vi "ief_read_data.vi"(0 "Tagprefix in":refnum<k21>, 11 "error in (no error)":errorcluster) -> (3 "PA Control Error":bool=TRUE, 4 "Tagprefix out":refnum<k21>, 6 "value real 32":sgl format="%.5f", 8 "value uint 32":u32, 10 "value uint 16":u16, 14 "PA Control state":u8, 15 "error out (no error)":errorcluster)   [LabVIEW 2015, in "IEF Werner.lvlib"]
doc: "This VI reads the input bytes from the IEF control and the PA status. \n\nNote that the tags of the DSC engine used by this VI have a strict name convention. This convention is described in the documentation of the VI tree.\n\nLicense Agreement for this software:\n\nCopyright (C)\nGesellschaft für Schwerionenforschung, GSI\nPlanckstr. 1\n64291 Darmstadt\nGermany\n\nContact: D.Beck@gsi.de \n\nThis program is free software; you can redistribute it and/or modify it under the terms of the \nGNU General Public License as published by the Free Software Foundation; either version 2 of \nthe license, or (at your option) any later version.\n\nThis program is distributed in the hope that it will be useful, but WITHOUT ANY WARRANTY; \nwithout even the implied warranty of MERCHANTABILITY or FITNESS FOR A PARTICULAR PURPOSE. See \nthe GNU General License for more details (http://www.gnu.org).\n\nGesellschaft für Schwerionenforschung, GSI\nPlanckstr. 1, 64291 Darmstadt, Germany\nFor all questions and ideas contact: M.Richter@gsi.de, H.Brand@gsi.de or D.Beck@gsi.de.\nLast update: 20-DEC-2002"
uses:
  IEF Werner.lvlib
  Packages/CSPP_Core/Libraries/Base/FGV Action.ctl
  <vilib>/lvdsc/legacy/tag/legacy_Read_Tag_(analog)7x.vi
  Packages/CSPP_Core/Libraries/Base/CS++Base.lvlib
panel:
  # "IEF Read Data"
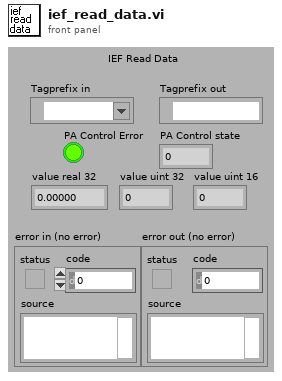
[diagram p1: front panel]
types:
  T1 = typedef "CS++Base.lvlib/FGV Action.ctl" = enum16{"add", "replace", "read", "remove", "reset", "get attributes"}
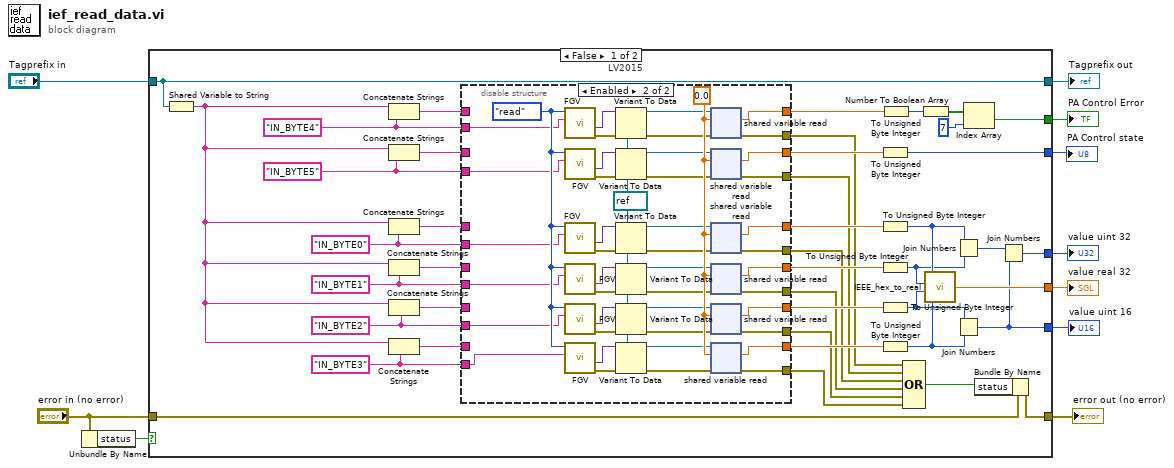
[diagram p0: block diagram]
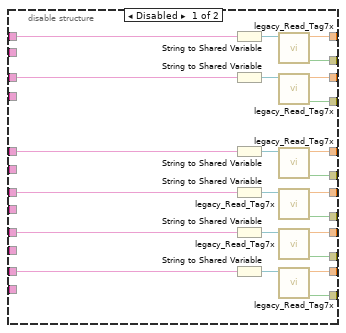
[diagram p2: hidden frame]
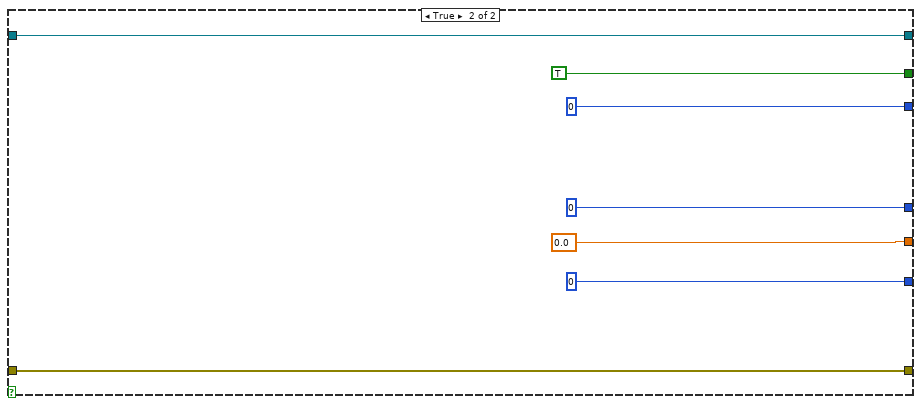
[diagram p3: hidden frame]
diagram:
  n1 = Unbundle By Name("error in (no error)") -> ("status"=w5:bool)
  n2 = case shown="False" w5 {
    tunnel: [w38 sgl 0.0 ("number 5")] -> w10
    tunnel: [w37 u32 0] -> w9
    tunnel: [w36 TRUE] -> w8
    tunnel: [w35 u8 0] -> w7
    tunnel: [w28 u16 0] -> w6
    tunnel: "error in (no error)" -> [w27 w123]
    tunnel: [w26 w123] -> w3
    tunnel: "Tagprefix in" -> [w17 w122]
    tunnel: [w17 w122] -> w1
    frame False {
      w11 = "IN_BYTE3" ("string")
      w12 = "IN_BYTE2" ("string")
      w13 = "IN_BYTE1" ("string")
      w14 = "IN_BYTE0" ("string")
      w15 = "IN_BYTE5"
      w16 = "IN_BYTE4"
      n3 = Shared Variable to String(1:w17) -> (0:w18:string)
      n4 = Concatenate Strings(w18, w16) -> (w24:string)
      n5 = Concatenate Strings(w18, w15) -> (w23:string)
      n6 = Concatenate Strings(w18, w14) -> (w22:string)
      n7 = Concatenate Strings(w18, w13) -> (w21:string)
      n8 = Concatenate Strings(w18, w12) -> (w20:string)
      n9 = Concatenate Strings(w18, w11) -> (w19:string)
      n10 = disable-structure "LV2015" shown="Enabled" {
        disable-tunnel: [w76 w111] -> w52
        disable-tunnel: [w75 w112] -> w51
        disable-tunnel: [w74 w113] -> w50
        disable-tunnel: [w73 w114] -> w49
        disable-tunnel: [w72 w109] -> w47
        disable-tunnel: [w71 w110] -> w43
        disable-tunnel: [w70 w116] -> w34
        disable-tunnel: [w69 w117] -> w33
        disable-tunnel: [w68 w118] -> w32
        disable-tunnel: [w67 w119] -> w31
        disable-tunnel: [w66 w121] -> w30
        disable-tunnel: [w65 w120] -> w29
        disable-tunnel: w24 -> [w58 _]
        disable-tunnel: w23 -> [w57 _]
        disable-tunnel: w22 -> [w56 _]
        disable-tunnel: w21 -> [w55 _]
        disable-tunnel: w20 -> [w54 _]
        disable-tunnel: w19 -> [w53 _]
        disable-tunnel: w16 -> [_ w82]
        disable-tunnel: w15 -> [_ w81]
        disable-tunnel: w14 -> [_ w80]
        disable-tunnel: w13 -> [_ w79]
        disable-tunnel: w12 -> [_ w78]
        disable-tunnel: w11 -> [_ w77]
        frame Disabled {
          n11 = String to Shared Variable(0:w58) -> (2:w64:refnum<k21>)  [unwired: 1 out]
          n12 = String to Shared Variable(0:w57) -> (2:w63:refnum<k21>)  [unwired: 1 out]
          n13 = String to Shared Variable(0:w56) -> (2:w62:refnum<k21>)  [unwired: 1 out]
          n14 = String to Shared Variable(0:w55) -> (2:w61:refnum<k21>)  [unwired: 1 out]
          n15 = String to Shared Variable(0:w54) -> (2:w60:refnum<k21>)  [unwired: 1 out]
          n16 = String to Shared Variable(0:w53) -> (2:w59:refnum<k21>)  [unwired: 1 out]
          n17 = call-poly <vilib>:"legacy_Read_Tag7x.vi"("tag name"=w64) -> ("error"=w65:bool, "value"=w72:dbl)  [unwired: 4 in, 5 out]
          n18 = call-poly <vilib>:"legacy_Read_Tag7x.vi"("tag name"=w63) -> ("error"=w66:bool, "value"=w71:dbl)  [unwired: 4 in, 5 out]
          n19 = call-poly <vilib>:"legacy_Read_Tag7x.vi"("tag name"=w62) -> ("error"=w67:bool, "value"=w76:dbl)  [unwired: 4 in, 5 out]
          n20 = call-poly <vilib>:"legacy_Read_Tag7x.vi"("tag name"=w61) -> ("error"=w68:bool, "value"=w75:dbl)  [unwired: 4 in, 5 out]
          n21 = call-poly <vilib>:"legacy_Read_Tag7x.vi"("tag name"=w60) -> ("error"=w69:bool, "value"=w74:dbl)  [unwired: 4 in, 5 out]
          n22 = call-poly <vilib>:"legacy_Read_Tag7x.vi"("tag name"=w59) -> ("error"=w70:bool, "value"=w73:dbl)  [unwired: 4 in, 5 out]
        }
        frame Enabled {
          w83 = FGV_Action."read" ("Action (read)")
          w96 = refnum<k21> refnum ("shared variable refnum in")
          w115 = 0.0
          n23 = call "FGV.vi"("Attribute Name"=w82, "Action (read)"=w83) -> ("Error Out"=w95:errorcluster, "Data out"=w89:variant)  [unwired: 5 in, 3 out]
          n24 = call "FGV.vi"("Attribute Name"=w81, "Action (read)"=w83) -> ("Error Out"=w90:errorcluster, "Data out"=w88:variant)  [unwired: 5 in, 3 out]
          n25 = call "FGV.vi"("Attribute Name"=w80, "Action (read)"=w83) -> ("Error Out"=w91:errorcluster, "Data out"=w87:variant)  [unwired: 5 in, 3 out]
          n26 = call "FGV.vi"("Attribute Name"=w79, "Action (read)"=w83) -> ("Error Out"=w92:errorcluster, "Data out"=w86:variant)  [unwired: 5 in, 3 out]
          n27 = call "FGV.vi"("Attribute Name"=w78, "Action (read)"=w83) -> ("Error Out"=w93:errorcluster, "Data out"=w85:variant)  [unwired: 5 in, 3 out]
          n28 = call "FGV.vi"("Attribute Name"=w77, "Action (read)"=w83) -> ("Error Out"=w94:errorcluster, "Data out"=w84:variant)  [unwired: 5 in, 3 out]
          n29 = Variant To Data(error in=w95, type=w96, Variant=w89) -> (data=w102:refnum<k21>, error out=w108:errorcluster)
          n30 = Variant To Data(error in=w90, type=w96, Variant=w88) -> (data=w101:refnum<k21>, error out=w107:errorcluster)
          n31 = Variant To Data(error in=w91, type=w96, Variant=w87) -> (data=w100:refnum<k21>, error out=w103:errorcluster)
          n32 = Variant To Data(error in=w92, type=w96, Variant=w86) -> (data=w99:refnum<k21>, error out=w104:errorcluster)
          n33 = Variant To Data(error in=w93, type=w96, Variant=w85) -> (data=w98:refnum<k21>, error out=w105:errorcluster)
          n34 = Variant To Data(error in=w94, type=w96, Variant=w84) -> (data=w97:refnum<k21>, error out=w106:errorcluster)
          n35 = shared-variable-read(w102, w108, w115) -> (w120:errorcluster, w109:dbl)  [unwired: 2 out]
          n36 = shared-variable-read(w101, w107, w115) -> (w121:errorcluster, w110:dbl)  [unwired: 2 out]
          n37 = shared-variable-read(w100, w103, w115) -> (w119:errorcluster, w111:dbl)  [unwired: 2 out]
          n38 = shared-variable-read(w99, w104, w115) -> (w118:errorcluster, w112:dbl)  [unwired: 2 out]
          n39 = shared-variable-read(w98, w105, w115) -> (w117:errorcluster, w113:dbl)  [unwired: 2 out]
          n40 = shared-variable-read(w97, w106, w115) -> (w116:errorcluster, w114:dbl)  [unwired: 2 out]
        }
      }
      n41 = To Unsigned Byte Integer(number=w43) -> (unsigned 8bit integer=w35:u8)
      n42 = To Unsigned Byte Integer(number=w52) -> (unsigned 8bit integer=w42:u8)
      n43 = To Unsigned Byte Integer(number=w51) -> (unsigned 8bit integer=w40:u8)
      n44 = To Unsigned Byte Integer(number=w50) -> (unsigned 8bit integer=w39:u8)
      n45 = To Unsigned Byte Integer(number=w49) -> (unsigned 8bit integer=w41:u8)
      n46 = To Unsigned Byte Integer(number=w47) -> (unsigned 8bit integer=w46:u8)
      n47 = Compound Arithmetic op=OR(w29, w30, w31, w32, w33, w34) -> (w25:bool)
      n48 = Number To Boolean Array(number=w46) -> (Boolean array=w45:bool[])
      n49 = call "IEEE_hex_to_real.vi"("number 4"=w41, "number 3"=w39, "number 2"=w40, "number"=w42) -> ("number 5"=w38:sgl)
      n50 = Join Numbers(hi=w42, lo=w40) -> ((hi.lo)=w48:u16)
      n51 = Join Numbers(hi=w39, lo=w41) -> ((hi.lo)=w28:u16)
      n52 = Index Array(array=w45, index=7 ("Index")) -> (element=w36:bool)
      n53 = Bundle By Name(cluster=w27, "status"=w25) -> (w26:errorcluster)
      n54 = Join Numbers(hi=w48, lo=w28) -> ((hi.lo)=w37:u32)
    }
    frame True {
    }
  }
  "value real 32" <- w10
  "value uint 32" <- w9
  "PA Control Error" <- w8
  "PA Control state" <- w7
  "value uint 16" <- w6
  "error out (no error)" <- w3
  "Tagprefix out" <- w1
